vi "Вывод записанной температуры.vi"() -> ()   [LabVIEW 2017]
doc: "This VI is used as a subVI in the Temperature System exercise in the LabVIEW Basics I course."
uses:
  <vilib>/Utility/file.llb/Read From Spreadsheet File (DBL).vi
panel:
  in  "Return":bool
  out "Температура":T1(graph)
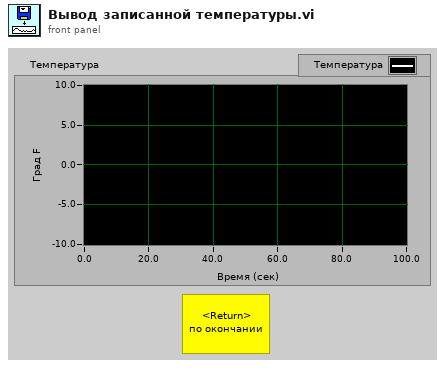
[diagram p1: front panel]
types:
  T1 = cluster{"Xo":i32, "Delta X":ext, "first row":dbl[]}
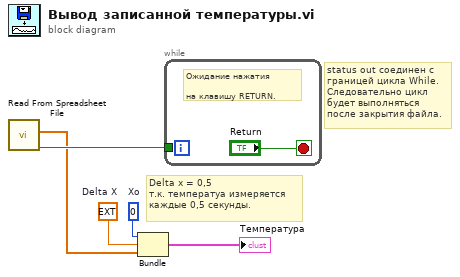
[diagram p0: block diagram]
diagram:
  w4 = ext 0.5  # Delta X
  w5 = 0  # Xo
  # "status out соединен с границей цикла While. Следовательно цикл будет выполняться после закрытия файла."
  # "Delta x = 0,5\nт.к. температуа измеряется \nкаждые 0,5 секунды."
  n1 = call-poly <vilib>:"Read From Spreadsheet File.vi"() -> ("EOF?"=w2:bool, "first row"=w1:dbl[])  [unwired: 7 in, 3 out]
  n2 = Bundle("Xo"=w5, "Delta X"=w4, "first row"=w1) -> (→"Температура":T1)  [unwired: 1 in]
  n3 = while {
    tunnel: w2 -> [_]
    stop <- "Return" stop-if-true
    # "Ожидание нажатия\n\nна клавишу RETURN."
  }
